vi "Ref to Address.vi"(10 "Reference":u32, 11 "Reference Format":u16(ring)=6 items=["4 Digits"=4, "5 Digits"=5, "6 Digits"=6]) -> (2 "Address":u16, 3 "Reference Type":T1=enum."Invalid")   [LabVIEW 2018, in "MB PLC Client.lvlib"]
uses:
  MB PLC Client.lvlib
  Types/Reference Types_Enum.ctl
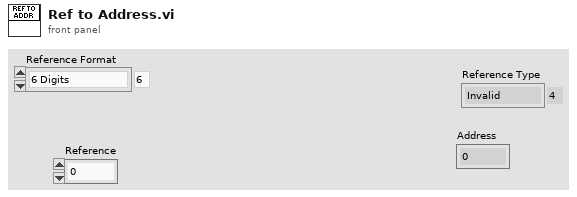
[diagram p1: front panel]
types:
  T1 = typedef "MB PLC Client.lvlib/Reference Types_Enum.ctl" = enum16{"Coil", "Discrete Input", "Input Register", "Holding Register", "Invalid"}
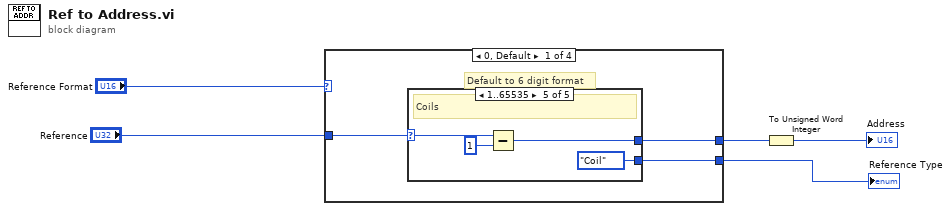
[diagram p0: block diagram]
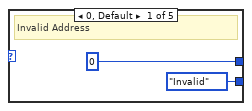
[diagram p2: hidden frame]
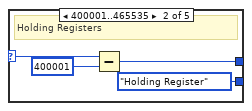
[diagram p3: hidden frame]
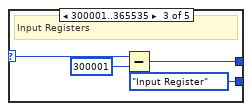
[diagram p4: hidden frame]
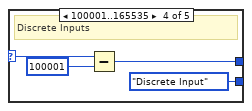
[diagram p5: hidden frame]
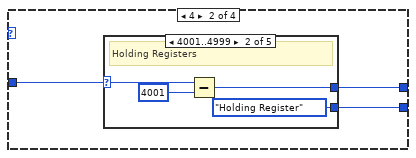
[diagram p6: hidden frame]
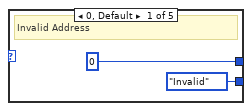
[diagram p7: hidden frame]
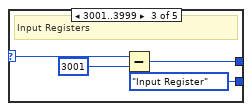
[diagram p8: hidden frame]
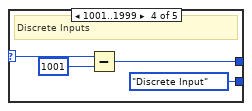
[diagram p9: hidden frame]
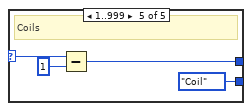
[diagram p10: hidden frame]
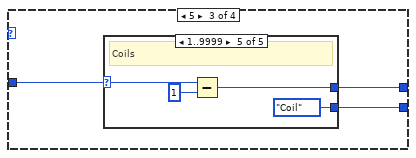
[diagram p11: hidden frame]
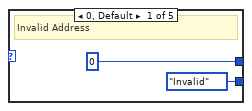
[diagram p12: hidden frame]
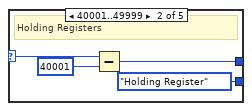
[diagram p13: hidden frame]
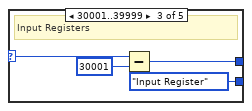
[diagram p14: hidden frame]
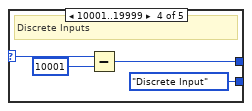
[diagram p15: hidden frame]
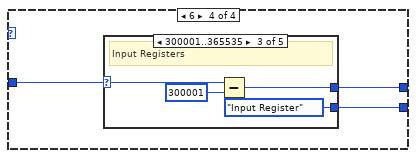
[diagram p16: hidden frame]
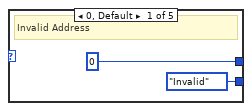
[diagram p17: hidden frame]
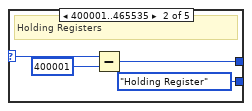
[diagram p18: hidden frame]
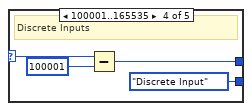
[diagram p19: hidden frame]
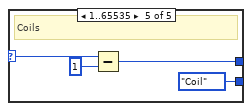
[diagram p20: hidden frame]
diagram:
  n1 = case shown="0, Default" "Reference Format" {
    tunnel: [w7 w29 w50 w71] -> w5
    tunnel: "Reference" -> [w8 w28 w48 w70]
    tunnel: [w6 w27 w49 w69] -> w2
    frame 0, Default {
      # "Default to 6 digit format"
      n2 = case shown="1..65535" w8 {
        selector: w8 -> [_ w14 w18 w21 w25]
        tunnel: [Reference_Types_Enum."Invalid" Reference_Types_Enum."Holding Register" Reference_Types_Enum."Input Register" Reference_Types_Enum."Discrete Input" Reference_Types_Enum."Coil"] -> w6
        tunnel: [u32 0 ("Address") w11 w17 w19 w23] -> w7
        frame 0, Default {
          # "Invalid Address"
        }
        frame 400001..465535 {
          # "Holding Registers"
          n3 = Subtract(x=w14, y=u32 400001 ("t")) -> (x-y=w11:u32)
        }
        frame 300001..365535 {
          # "Input Registers"
          n4 = Subtract(x=w18, y=u32 300001) -> (x-y=w17:u32)
        }
        frame 100001..165535 {
          # "Discrete Inputs"
          n5 = Subtract(x=w21, y=u32 100001 ("t")) -> (x-y=w19:u32)
        }
        frame 1..65535 {
          # "Coils"
          n6 = Subtract(x=w25, y=u32 1) -> (x-y=w23:u32)
        }
      }
    }
    frame 4 {
      n7 = case shown="4001..4999" w28 {
        selector: w28 -> [_ w35 w39 w42 w46]
        tunnel: [Reference_Types_Enum."Invalid" Reference_Types_Enum."Holding Register" Reference_Types_Enum."Input Register" Reference_Types_Enum."Discrete Input" Reference_Types_Enum."Coil"] -> w27
        tunnel: [u32 0 ("Address") w32 w38 w40 w44] -> w29
        frame 0, Default {
          # "Invalid Address"
        }
        frame 4001..4999 {
          # "Holding Registers"
          n8 = Subtract(x=w35, y=u32 4001 ("t")) -> (x-y=w32:u32)
        }
        frame 3001..3999 {
          # "Input Registers"
          n9 = Subtract(x=w39, y=u32 3001) -> (x-y=w38:u32)
        }
        frame 1001..1999 {
          # "Discrete Inputs"
          n10 = Subtract(x=w42, y=u32 1001 ("t")) -> (x-y=w40:u32)
        }
        frame 1..999 {
          # "Coils"
          n11 = Subtract(x=w46, y=u32 1) -> (x-y=w44:u32)
        }
      }
    }
    frame 5 {
      n12 = case shown="1..9999" w48 {
        selector: w48 -> [_ w56 w60 w63 w67]
        tunnel: [Reference_Types_Enum."Invalid" Reference_Types_Enum."Holding Register" Reference_Types_Enum."Input Register" Reference_Types_Enum."Discrete Input" Reference_Types_Enum."Coil"] -> w49
        tunnel: [u32 0 ("Address") w53 w59 w61 w65] -> w50
        frame 0, Default {
          # "Invalid Address"
        }
        frame 40001..49999 {
          # "Holding Registers"
          n13 = Subtract(x=w56, y=u32 40001 ("t")) -> (x-y=w53:u32)
        }
        frame 30001..39999 {
          # "Input Registers"
          n14 = Subtract(x=w60, y=u32 30001) -> (x-y=w59:u32)
        }
        frame 10001..19999 {
          # "Discrete Inputs"
          n15 = Subtract(x=w63, y=u32 10001 ("t")) -> (x-y=w61:u32)
        }
        frame 1..9999 {
          # "Coils"
          n16 = Subtract(x=w67, y=u32 1) -> (x-y=w65:u32)
        }
      }
    }
    frame 6 {
      n17 = case shown="300001..365535" w70 {
        selector: w70 -> [_ w77 w81 w84 w88]
        tunnel: [Reference_Types_Enum."Invalid" Reference_Types_Enum."Holding Register" Reference_Types_Enum."Input Register" Reference_Types_Enum."Discrete Input" Reference_Types_Enum."Coil"] -> w69
        tunnel: [u32 0 ("Address") w74 w80 w82 w86] -> w71
        frame 0, Default {
          # "Invalid Address"
        }
        frame 400001..465535 {
          # "Holding Registers"
          n18 = Subtract(x=w77, y=u32 400001 ("t")) -> (x-y=w74:u32)
        }
        frame 300001..365535 {
          # "Input Registers"
          n19 = Subtract(x=w81, y=u32 300001) -> (x-y=w80:u32)
        }
        frame 100001..165535 {
          # "Discrete Inputs"
          n20 = Subtract(x=w84, y=u32 100001 ("t")) -> (x-y=w82:u32)
        }
        frame 1..65535 {
          # "Coils"
          n21 = Subtract(x=w88, y=u32 1) -> (x-y=w86:u32)
        }
      }
    }
  }
  "Reference Type" <- w2
  n22 = To Unsigned Word Integer(number=w5) -> (unsigned 16bit integer=→"Address":u16)
